vi "Read from Excel file (old).vi"(7 "sheetname (\"\") - leave blank for first sheet":string, 8 "error in (no error)":errorcluster, 11 "File Name":path=path "C:/PhaeronGit/LVNPOI/Scratch/test.xls") -> (0 "error out":errorcluster, 2 "Values":string[][](array[string]))   [LabVIEW 2013]
doc: "Writes the 2D string array to the named Excel format file."
uses:
  Data/Polymorphic VIs/Get Cells (2D Row Part String).vi
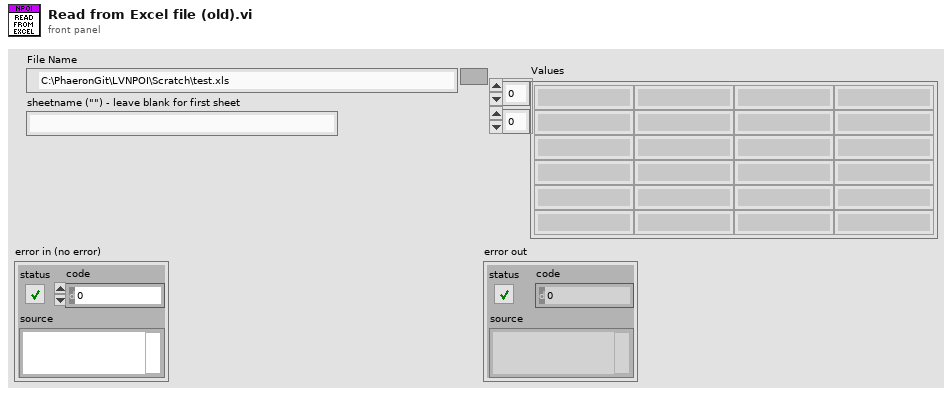
[diagram p1: front panel]
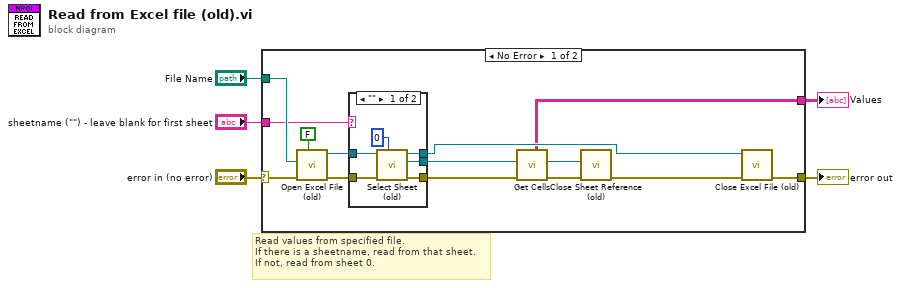
[diagram p0: block diagram]
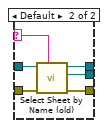
[diagram p2: hidden frame]
diagram:
  # "Read values from specified file.\nIf there is a sheetname, read from that sheet.\nIf not, read from sheet 0."
  n1 = case shown="No Error" "error in (no error)" {
    selector: "error in (no error)" -> [w18 w32]
    tunnel: "File Name" -> [w17 _]
    tunnel: "sheetname (\"\") - leave blank for first sheet" -> [w13 _]
    tunnel: [w19 w32] -> w3
    tunnel: [w6 _] -> w1
    frame No Error {
      n2 = call "Open Excel File (old).vi"(7:FALSE ("Create if does not exist? (T)"), "error in (no error)"=w18, "File Name"=w17) -> ("error out"=w15:errorcluster, "IWorkbook Reference Out"=w14:refnum<k24>)  [unwired: 7 in]
      n3 = case shown="\"\"" w13 {
        selector: w13 -> [_ w29]
        tunnel: w15 -> [w25 w31]
        tunnel: w14 -> [w24 w30]
        tunnel: [w22 w28] -> w7
        tunnel: [w21 w27] -> w11
        tunnel: [w20 w26] -> w12
        frame "" {
          n4 = call "Select Sheet (old).vi"("Sheet"=0, "error in (no error)"=w25, "Workbook Reference"=w24) -> ("error out"=w20:errorcluster, "Sheet Reference"=w21:refnum<k24>, "Workbook Reference"=w22:refnum<k24>)  [unwired: 6 in]
        }
        frame Default {
          n5 = call "Select Sheet by Name (old).vi"("Sheet (Sheet1)"=w29, "error in (no error)"=w31, "Workbook Reference"=w30) -> ("error out"=w26:errorcluster, "Sheet Reference"=w27:refnum<k24>, "Workbook Reference"=w28:refnum<k24>)  [unwired: 6 in]
        }
      }
      n6 = call-poly "Get Cells.vi"("error in (no error)"=w12, "Sheet Reference"=w11) -> ("error out"=w10:errorcluster, "Sheet Reference out"=w9:refnum<k24>, "Values"=w6:string[][])  [unwired: 7 in]
      n7 = call "Close Sheet Reference (old).vi"("error in (no error)"=w10, "Sheet Reference"=w9) -> ("error out"=w8:errorcluster)  [unwired: 9 in]
      n8 = call "Close Excel File (old).vi"("error in (no error)"=w8, "IWorkbook Reference"=w7) -> ("error out"=w19:errorcluster)  [unwired: 9 in]
    }
    frame Error {
    }
  }
  "error out" <- w3
  "Values" <- w1
